vi "Read Exception Status.vi"(8 "error in (no error)":errorcluster, 11 "Modbus master in":refnum<class "Network Master.lvclass">) -> (0 "error out":errorcluster, 2 "exception status":u8, 3 "Modbus master out":refnum<class "Network Master.lvclass">)   [LabVIEW 2021, in "Network Master.lvclass"]
doc: "Reads the exception status of a Modbus slave. The exception status is a set of eight status bits. Each status bit represents an exception."
uses:
  Network Master.lvclass
  D:/my_projects/projects/Algorithms/Labview/21/Modbus_v121c/Network Protocol/Network Protocol.lvclass
  Serial/Serial Master.lvclass
  Modbus Data Unit/Modbus Data Unit.lvclass/Modbus Data Unit.ctl
  Network Protocol.lvclass/Network Protocol.ctl
  Network Master.lvclass/Network Master.ctl
  Modbus Data Unit/Construct PDU.vi
  Data Model/Error Generator.vi
  Master Function Definition/Function code mismatch error.vi
  Modbus Data Unit/Deconstruct PDU.vi
  Read Transmission Data Unit.vi
  Modbus Data Unit/Modbus Data Unit.lvclass
  Transmission Data Unit/Transmission Data Unit.lvclass
  Master Function Definition/Master Function Definition.lvclass
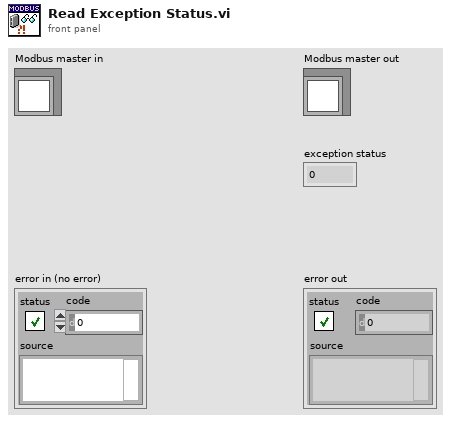
[diagram p1: front panel]
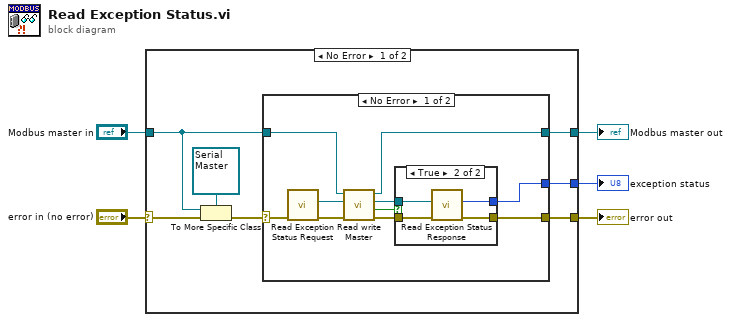
[diagram p0: block diagram]
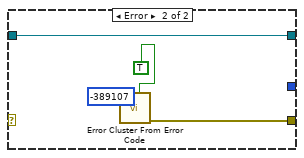
[diagram p3: hidden frame]
diagram:
  n1 = case shown="No Error" "error in (no error)" {
    selector: "error in (no error)" -> [w8 w32]
    tunnel: [w12 w33] -> w5
    tunnel: "Modbus master in" -> [w7 w33]
    tunnel: [w11 _] -> w3
    tunnel: [w10 w32] -> w2
    frame No Error {
      n2 = To More Specific Class(target class=refnum<class "Serial Master.lvclass"> refnum ("Serial Master"), reference=w7, error in=w8) -> (error out=w9:errorcluster)  [unwired: 1 out]
      n3 = case shown="No Error" w9 {
        selector: w9 -> [w18 _]
        tunnel: w7 -> [w13 w30]
        tunnel: [w14 w30] -> w12
        tunnel: [w21 _] -> w11
        tunnel: [w19 w31] -> w10
        frame No Error {
          n4 = call "Read Exception Status Request.vi"("error in"=w18) -> ("error out"=w22:errorcluster, "modbus data unit out"=w17:refnum<class "Modbus Data Unit.lvclass">)  [unwired: 9 in]
          n5 = call "Read write Master.vi"("error in (no error)"=w22, "Modbus data unit in"=w17, "Modbus master in"=w13) -> ("error out"=w20:errorcluster, "PDU valid?"=w16:bool, "Modbus data unit out"=w15:refnum<class "Modbus Data Unit.lvclass">, "Modbus master out"=w14:refnum<class "Network Master.lvclass">)  [unwired: 5 in]
          n6 = case shown="True" w16 {
            tunnel: [_ w27] -> w21
            tunnel: w15 -> [_ w26]
            tunnel: w20 -> [w23 w25]
            tunnel: [w23 w24] -> w19
            frame False {
            }
            frame True {
              n7 = call "Read Exception Status Response.vi"("error in"=w25, "modbus data unit in"=w26) -> ("error out"=w24:errorcluster, "Exception Status"=w27:u8)  [unwired: 8 in]
            }
          }
        }
        frame Error {
          n8 = call <vilib>:"Error Cluster From Error Code.vi"("is warning? (False)"=TRUE, "error code (0)"=-389107) -> ("error out"=w31:errorcluster)  [unwired: 7 in]
        }
      }
    }
    frame Error {
    }
  }
  "error out" <- w2
  "Modbus master out" <- w5
  "exception status" <- w3
